vi "lowpass location estimate.vi"(10 "axis number":u8=2, 11 "kalman state":T1) -> (3 "location":i16)   [LabVIEW 2010]
uses:
  integrating single axis kalman state.ctl
  <vilib>/rvi/Analysis/common/polyVINode/niFpgaPolyViWrapper.xnode
  <vilib>/express/rvi/analysis/control/discrete linear/niFPGA Discrete Control Filter.vi
panel:
  out "z state.pos estimate":fxp<+/-,32,16> format="%.21g"
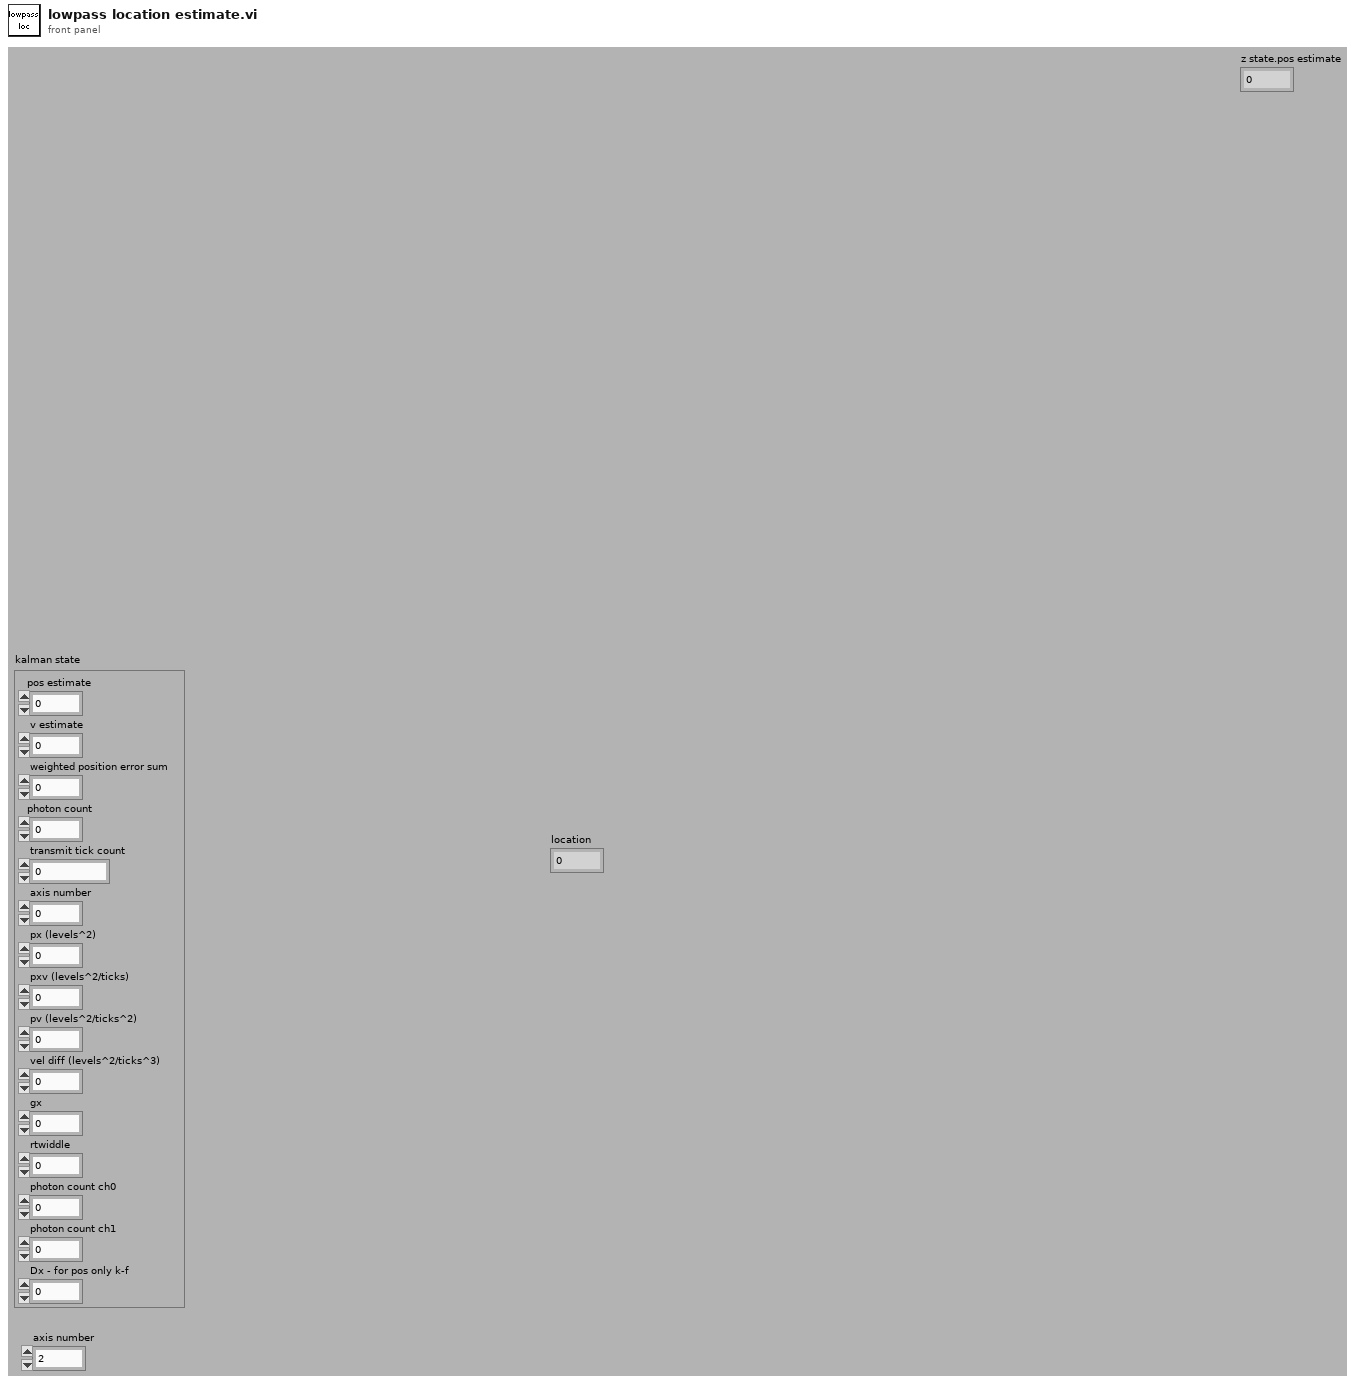
[diagram p1: front panel]
types:
  T1 = typedef "integrating single axis kalman state.ctl" = cluster{"pos estimate":fxp<+/-,32,16>, "v estimate":fxp<+/-,16,0>, "weighted position error sum":fxp<+/-,32,32>, "photon count":u32, "transmit tick count":u32, "axis number":u8, "px (levels^2)":fxp<+,32,19>, "pxv (levels^2/ticks)":fxp<+,32,2>, "pv (levels^2/ticks^2)":fxp<+,32,-14>, "vel diff (levels^2/ticks^3)":fxp<+,24,-22>, "gx":fxp<+,16,8>, "rtwiddle":fxp<+,16,26>, "photon count ch0":u32, "photon count ch1":u32, "Dx - for pos only k-f":fxp<+,32,19>}
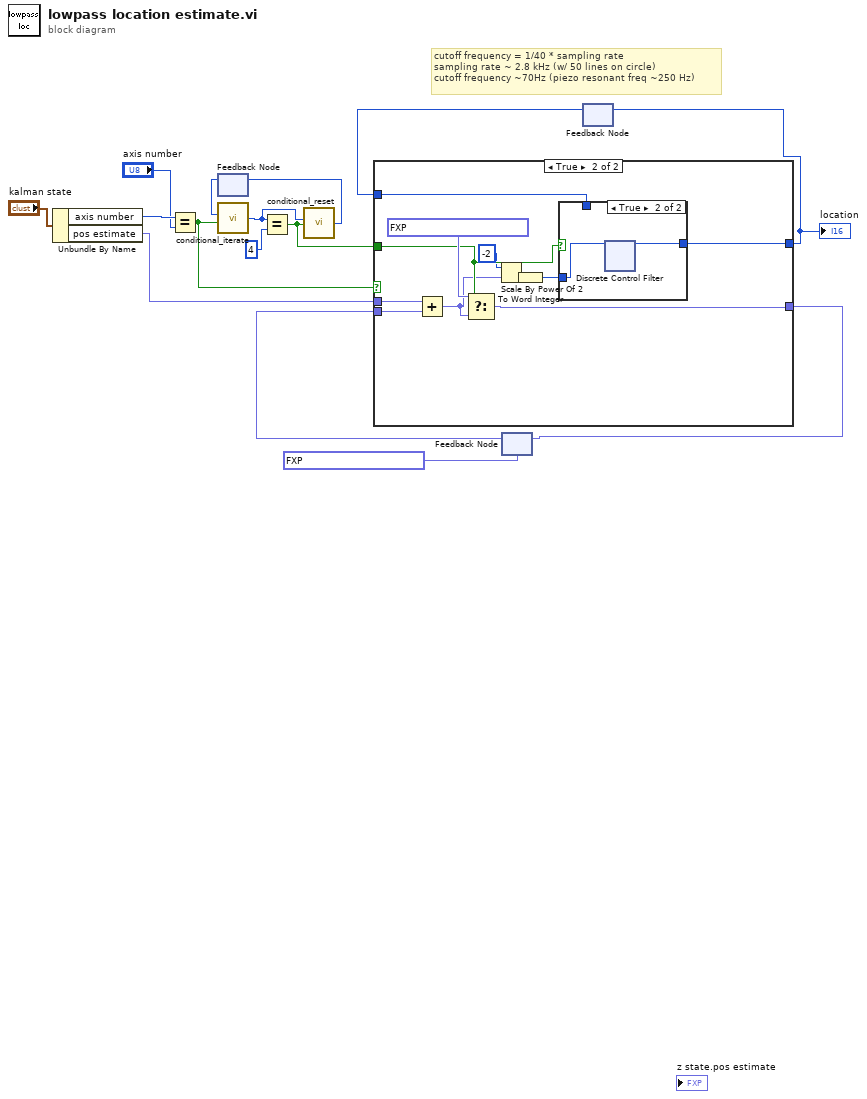
[diagram p0: block diagram]
diagram:
  # "cutoff frequency = 1/40 * sampling rate\nsampling rate ~ 2.8 kHz (w/ 50 lines on circle)\ncutoff frequency ~70Hz (piezo resonant freq ~250 Hz)"
  n1 = Unbundle By Name("kalman state") -> ("axis number"=w14:u8, "pos estimate"=w6:fxp<+/-,32,16>)
  n2 = Equal?(x=w14, y="axis number") -> (x = y?=w8:bool)
  n3 = feedback #1() -> (w12:u16)  [unwired: 1 in]
  n4 = call "conditional_iterate.vi"("iterate?"=w8, "number in"=w12) -> ("number out"=w10:u16)  [unwired: 4 in]
  n5 = Equal?(x=w10, y=u16 4) -> (x = y?=w7:bool)
  n6 = call "conditional_reset.vi"("reset?"=w7, "number in"=w10) -> ("number out"=w9:u16)  [unwired: 4 in]
  n7 = feedback-in #1(w9) -> ()
  n8 = feedback #2(fxp<+/-,32,16> 0.0 ("pos estimate")) -> (w5:fxp<+/-,34,18>)
  n9 = feedback #3() -> (w1:i16)  [unwired: 1 in]
  n10 = case shown="True" w8 {
    tunnel: w7 -> [_ w24]
    tunnel: w6 -> [_ w28]
    tunnel: [w16 w25] -> w3
    tunnel: w5 -> [w16 w27]
    tunnel: [w17 w19] -> w2
    tunnel: w1 -> [w17 w18]
    frame False {
    }
    frame True {
      n11 = Add(x=w28, y=w27) -> (x+y=w23:fxp<+/-,34,18>)
      n12 = Select(t=fxp<+/-,32,16> 0.0 ("pos estimate"), s=w24, f=w23) -> (s? t:f=w25:fxp<+/-,34,18>)
      n13 = Scale By Power Of 2(n=-2, x=w23) -> (x*2^n=w22:fxp<+/-,34,18>)
      n14 = To Word Integer(number=w22) -> (16bit integer=w20:i16)
      n15 = case shown="True" w24 {
        tunnel: w20 -> [_ w31]
        tunnel: [w29 w30] -> w19
        tunnel: w18 -> [w29 _]
        frame False {
        }
        frame True {
          n16 = xnode ("Discrete Control Filter")("input"=w31) -> ("output"=w30:i16)  [unwired: 1 in]
        }
      }
    }
  }
  "location" <- w2
  n17 = feedback-in #2(w3) -> ()
  n18 = feedback-in #3(w2) -> ()
